vi "lib return error.vi"(8 "error in":errorcluster, 11 "return value":i32) -> (0 "error out":errorcluster)   [LabVIEW 2013, in "Shared Library Module runtime.lvclass"]
uses:
  Shared Library Module runtime.lvclass
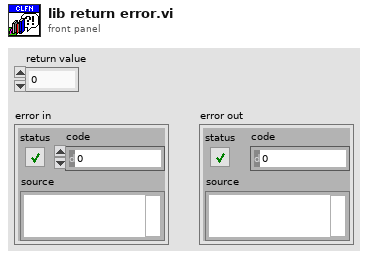
[diagram p1: front panel]
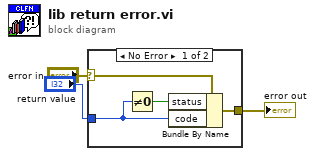
[diagram p0: block diagram]
diagram:
  n1 = case shown="No Error" "error in" {
    selector: "error in" -> [w7 w8]
    tunnel: "return value" -> [w6 _]
    tunnel: [w4 w8] -> w3
    frame No Error {
      n2 = Not Equal To 0?(x=w6) -> (x != 0?=w5:bool)
      n3 = Bundle By Name(cluster=w7, "status"=w5, "code"=w6) -> (w4:errorcluster)
    }
    frame Error {
    }
  }
  "error out" <- w3
